vi "MathCad_Easy_Numeric_Get_Multiple_Var.vi"(8 "error in (no error)":errorcluster, 10 "Array of Names":string[](array[string]), 11 "Mathcad Reference":T1) -> (0 "error out":errorcluster, 2 "Data Out":T2(array[cluster]) {"value" format="%.2f"}, 3 "Mathcad Reference":T1)   [LabVIEW 2015]
doc: "Gets the numeric value in Mathcad. It gets the last definition of the variable.\n\nInputs\n Wrksht Ref--ActiveX Reference to Mathcad Worksheet Class\n Array of Names (Array of Strings)\n\nOutputs\n Wrksht Ref--ActiveX Reference to Mathcad Worksheet Class \n Data Out(Array of Clusters)\n Cluster(2 Elements) \n Variable Name (string)- Name of the new variable to be retrieved.\n Value(Double)- Value of last definition of variable in worksheet."
uses:
  Mathcad Reference.ctl
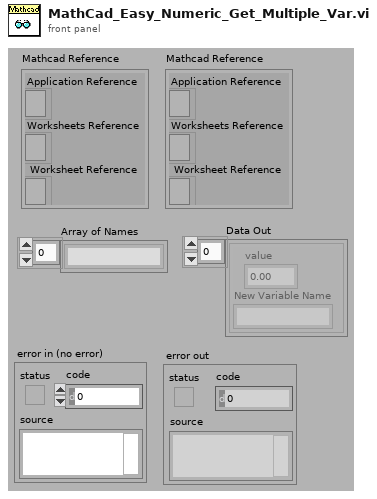
[diagram p1: front panel]
types:
  T1 = typedef "Mathcad Reference.ctl" = cluster{"Application Reference":refnum<k7>, "Worksheets Reference":refnum<k7>, " Worksheet Reference":refnum<k7>}
  T2 = cluster{"value":dbl, "New Variable Name":string}[]
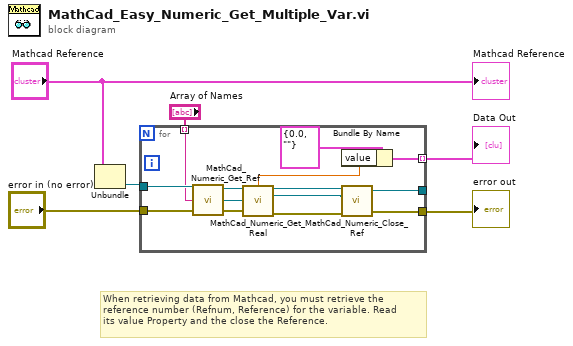
[diagram p0: block diagram]
diagram:
  # "When retrieving data from Mathcad, you must retrieve the \nreference number (Refnum, Reference) for the variable. Read \nits value Property and the close the Reference."
  n1 = Unbundle("Mathcad Reference") -> ("Worksheet Reference"=w3:refnum<k7>)  [unwired: 2 out]
  n2 = for {
    tunnel: "Array of Names" -> [w8] mode=indexing
    tunnel: "error in (no error)" -> [w19]
    tunnel: w3 -> [w20]
    tunnel: [w15] -> w1 mode=indexing
    tunnel: [w13] -> w4
    tunnel: [w10] -> _
    n3 = call "MathCad_Numeric_Get_Ref.vi"("error in (no error)"=w19, "Variable  Name"=w8, "Worksheet Reference In"=w20) -> ("error out"=w16:errorcluster, "Mathcad.INumericValue Refnum"=w17:refnum<k7>, "Worksheet Reference Out"=w18:refnum<k7>)
    n4 = call "MathCad_Numeric_Get_Real.vi"("Worksheet Reference In"=w18, "Mathcad.INumericValue Refnum In"=w17, "error in"=w16) -> ("value"=w9:dbl, "Worksheet Reference Out"=w12:refnum<k7>, "Mathcad.INumericValue Refnum Out"=w11:refnum<k7>, "error out"=w14:errorcluster)  [unwired: 9 in]
    n5 = Bundle By Name(cluster=cluster{"value":dbl, "New Variable Name":string} {"value"=0.0, "New Variable Name"=""}, "value"=w9) -> (w15:cluster{"value":dbl, "New Variable Name":string})
    n6 = call "MathCad_Numeric_Close_Ref.vi"("error in"=w14, "Mathcad.INumericValue Reference"=w11, "IMathcadWorksheet Reference"=w12) -> ("error out"=w13:errorcluster, "IMathcadWorksheet Reference"=w10:refnum<k7>)  [unwired: 2 in]
  }
  "error out" <- w4
  "Data Out" <- w1
  "Mathcad Reference" <- "Mathcad Reference"
